vi "getDeviceStatus.vi"(8 "error in (no error)":errorcluster, 11 "domeCommunicator in":refnum<class "DomeCommunicator.lvclass">) -> (0 "error out":errorcluster, 2 "status":T1, 3 "domeCommunicator out":refnum<class "DomeCommunicator.lvclass">)   [LabVIEW 2016, in "DomeCommunicator.lvclass"]
uses:
  DomeCommunicator.lvclass
  common_labview_tcpdevice/typedefs/deviceStatus.ctl
  common_labview_tcpdevice/typedefs/statusEnum.ctl
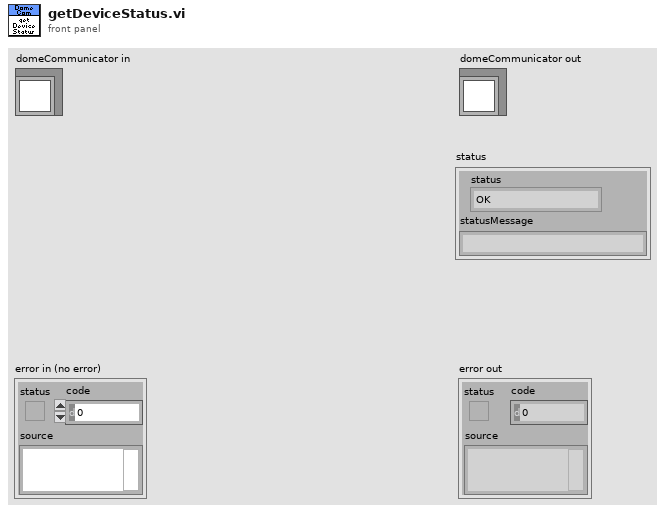
[diagram p1: front panel]
types:
  T1 = typedef "deviceStatus.ctl" = cluster{"status":T2, "statusMessage":string}
  T2 = typedef "statusEnum.ctl" = enum16{"OK", "TIMEOUT", "MSGERROR"}
  T3 = typedef "shortStatus.ctl" = cluster{"mainDoor":T4, "mainDoorOpeningPercentage":T5, "dropoutDoor":T4, "dropoutDoorOpeningPercentage":T5, "autoShutdownOn":bool, "sensorCode":T6, "domePosition":T7, "azimuthAngle":T8, "LastRotationDirection":T9, "state":T10}
  T4 = typedef "openingStates.ctl" = enum16{"Open", "Shut", "Ajar"}
  T5 = typedef "openingPercentage.ctl" = dbl
  T6 = typedef "sensorCode.ctl" = enum16{"None", "RainSnowSensorTriggered", "CloudSensorTriggered", "BothSensorsTriggered"}
  T7 = typedef "azimimuthPositionStatus.ctl" = enum16{"NotInHome", "Home"}
  T8 = typedef "azimuth.ctl" = dbl
  T9 = typedef "direction.ctl" = enum16{"ClockWise", "CounterClockWise"}
  T10 = typedef "domeState.ctl" = cluster{"azimuthMotion":T11, "mainDoorMotion":T12, "dropoutDoorMotion ":T12, "seekingHome":bool, "emergencyStopActivated":bool}
  T11 = typedef "motionDirection.ctl" = enum16{"NoMotion", "MovingClockWise", "MovingCounterClockWise"}
  T12 = typedef "openingMotion.ctl" = enum16{"NoMotion", "Opening", "Closing"}
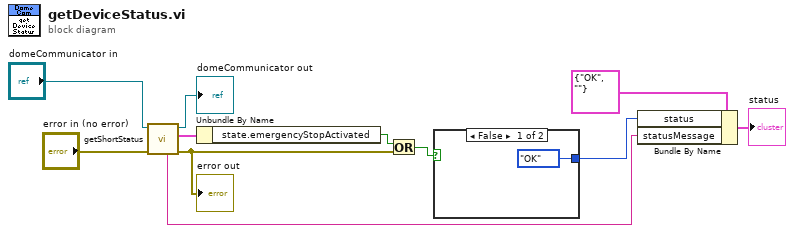
[diagram p0: block diagram]
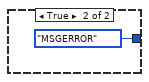
[diagram p2: hidden frame]
diagram:
  n1 = call "getShortStatus.vi"("error in (no error)"="error in (no error)", "DomeCommunicator in"="domeCommunicator in") -> ("error out"=w6:errorcluster, "shortStatus out"=w8:T3, "DomeCommunicator out"=→"domeCommunicator out":refnum<class "DomeCommunicator.lvclass">, "response"=w2:string)  [unwired: 5 in, 1 out]
  "error out" <- w6
  n2 = Unbundle By Name(w8) -> ("state.emergencyStopActivated"=w7:bool)
  n3 = Or(x=w7, y=w6) -> (x .or. y?=w5:bool)
  n4 = case shown="False" w5 {
    tunnel: [statusEnum."OK" ("status") statusEnum."MSGERROR" ("status")] -> w3
    frame False {
    }
    frame True {
    }
  }
  n5 = Bundle By Name(cluster=T1 {"status"=enum."OK", "statusMessage"=""} ("status"), "status"=w3, "statusMessage"=w2) -> (→"status":T1)
